vi "sc5511a_close_device.vi"(0 "deviceHandle":u32 format="%.0x", 5 "error in (no error)":errorcluster) -> (19 "error out":errorcluster)   [LabVIEW 2010]
uses:
  sc5511a.dll
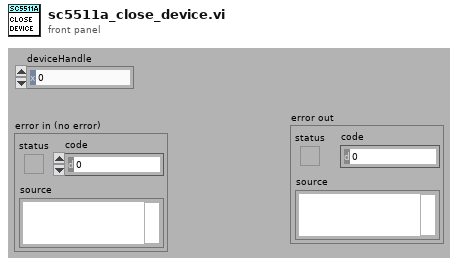
[diagram p1: front panel]
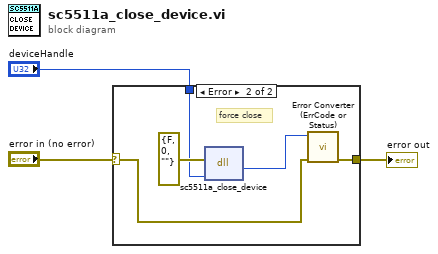
[diagram p0: block diagram]
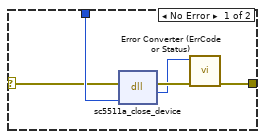
[diagram p2: hidden frame]
diagram:
  n1 = case shown="Error" "error in (no error)" {
    selector: "error in (no error)" -> [w4 w12]
    tunnel: [w8 w11] -> w2
    tunnel: "deviceHandle" -> [w6 w9]
    frame No Error {
      n2 = dll-call lib="sc5511a.dll" fn="sc5511a_close_device"(error in=w4, "deviceHandle"=w6) -> (error out=w7:errorcluster, "return type"=w5:i32)  [unwired: 3 in, 1 out]
      n3 = call "Error Converter (ErrCode or Status).vi"("error in (no error)"=w7, "error code"=w5) -> ("error out"=w8:errorcluster)  [unwired: 9 in]
    }
    frame Error {
      # "force close"
      n4 = dll-call lib="sc5511a.dll" fn="sc5511a_close_device"(error in=errorcluster {"status"=FALSE, "code"=0, "source"=""} ("error in (no error)"), "deviceHandle"=w9) -> ("return type"=w13:i32)  [unwired: 3 in, 2 out]
      n5 = call "Error Converter (ErrCode or Status).vi"("error in (no error)"=w12, "error code"=w13) -> ("error out"=w11:errorcluster)  [unwired: 9 in]
    }
  }
  "error out" <- w2
